vi "get_scan_input_meta_data.vi"(8 "error in":errorcluster, 11 "Path":path) -> (0 "error out":errorcluster, 2 "fpga_input":dbl[](array[numeric]), 3 "meta_data":T1)   [LabVIEW 2017]
uses:
  controls/scan_input_meta_data.ctl
  controls/scan-mode-CTL.ctl
panel:
  in  "type-cluster":T3
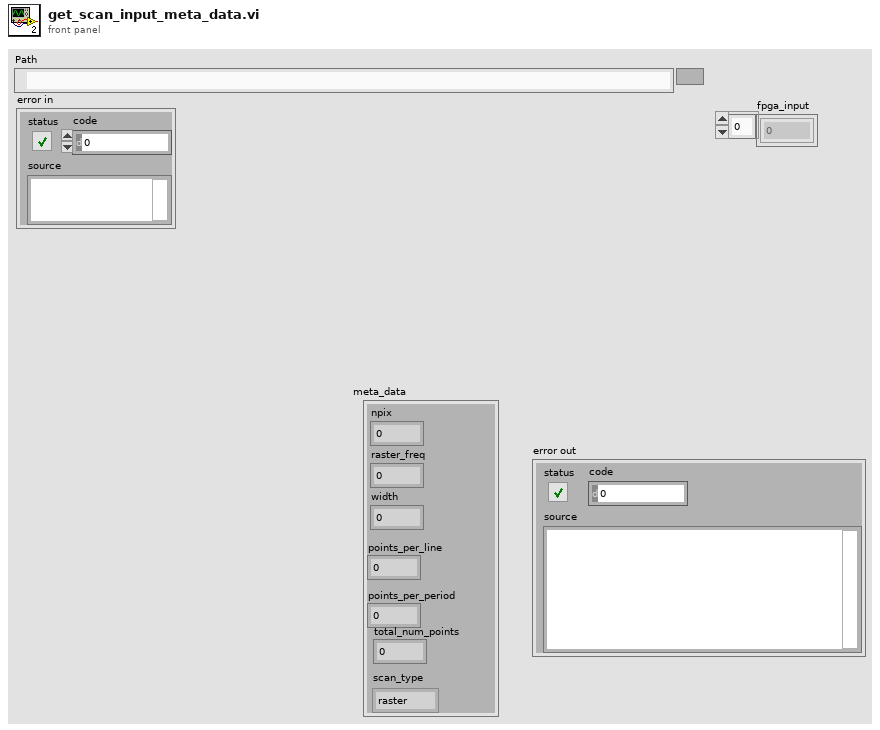
[diagram p1: front panel]
types:
  T1 = typedef "scan_input_meta_data.ctl" = cluster{"npix":i64, "raster_freq":dbl, "width":dbl, "points_per_line":i64, "points_per_period":i64, "total_num_points":i64, "scan_type":T2}
  T2 = typedef "scan-mode-CTL.ctl" = enum16{"raster", "CS"}
  T3 = cluster{"fpga_input":dbl[], "npix":i64, "raster_freq":dbl, "width":dbl, "points_per_line":i64, "points_per_period":i64, "total_num_points":i64, "scan_type":i64}
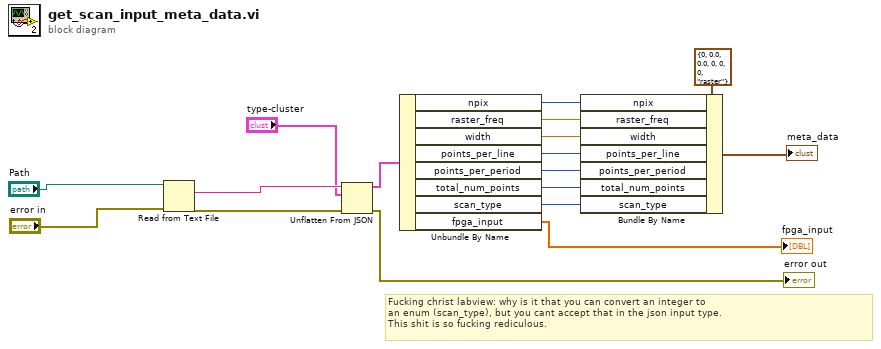
[diagram p0: block diagram]
diagram:
  # "Fucking christ labview: why is it that you can convert an integer to\nan enum (scan_type), but you cant accept that in the json input type.\nThis shit is so fucking rediculous."
  n1 = Read from Text File(file (use dialog)="Path", error in="error in") -> (text=w13:string, error out=w15:errorcluster)  [unwired: 2 in, 2 out]
  n2 = Unflatten From JSON(JSON string=w13, type and defaults="type-cluster", error in (no error)=w15) -> (value=w1:T3, error out=→"error out":errorcluster)  [unwired: 4 in]
  n3 = Unbundle By Name(w1) -> ("npix"=w11:i64, "raster_freq"=w10:dbl, "width"=w9:dbl, "points_per_line"=w8:i64, "points_per_period"=w7:i64, "total_num_points"=w6:i64, "scan_type"=w5:i64, "fpga_input"=→"fpga_input":dbl[])
  n4 = Bundle By Name(cluster=T1 {"npix"=0, "raster_freq"=0.0, "width"=0.0, "points_per_line"=0, "points_per_period"=0, "total_num_points"=0, "scan_type"=enum."raster"} ("value 2"), "npix"=w11, "raster_freq"=w10, "width"=w9, "points_per_line"=w8, "points_per_period"=w7, "total_num_points"=w6, "scan_type"=w5) -> (→"meta_data":T1)
